vi "Decode Error.vi"(8 "Error In":errorcluster) -> (3 "Status Message":string="Invalid XNET Interface")   [LabVIEW 2025, in "Automotive Ethernet Bus Monitor.lvclass"]
uses:
  Automotive Ethernet Bus Monitor.lvclass
  Automotive Ethernet Bus Monitor.lvclass/Automotive Ethernet Bus Monitor.ctl
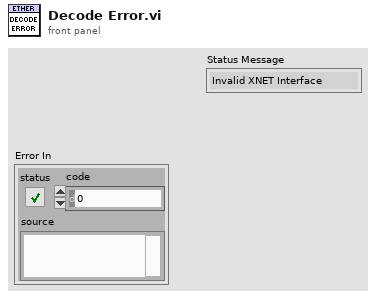
[diagram p1: front panel]
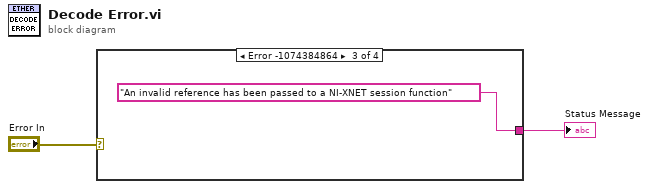
[diagram p0: block diagram]
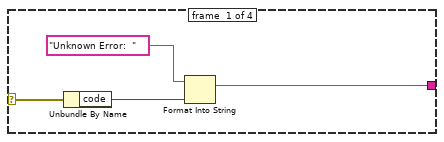
[diagram p2: hidden frame]
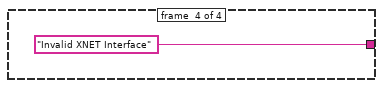
[diagram p4: hidden frame]
diagram:
  n1 = case shown="Error -1074384864" "Error In" {
    selector: "Error In" -> [w6 _ _ _]
    tunnel: [w5 _ "An invalid reference has been passed to a NI-XNET session function" "Invalid XNET Interface"] -> w2
    frame #0 {
      n2 = Unbundle By Name(w6) -> ("code"=w4:i32)
      n3 = Format Into String(initial string="Unknown Error:  ", w4) -> (resulting string=w5:string)  [unwired: 2 in, 1 out]
    }
    frame #1 {
    }
    frame #2 {
    }
    frame #3 {
    }
  }
  "Status Message" <- w2
